vi "PointsToROI.vi"(11 "Points":dbl[][](array[numeric])) -> (3 "ROIs":T1(array[cluster]))   [LabVIEW 2012]
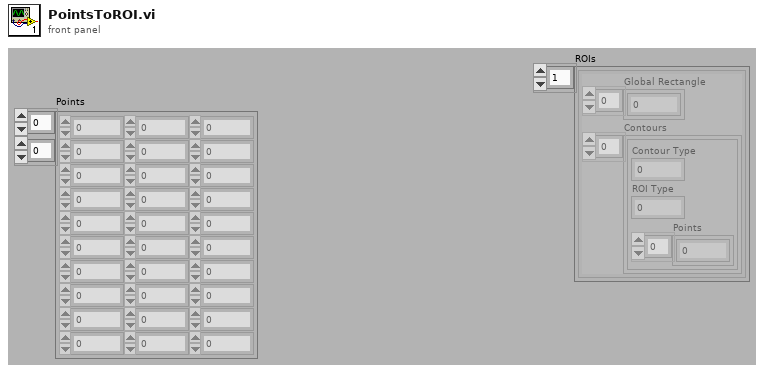
[diagram p1: front panel]
types:
  T1 = cluster{"Global Rectangle":i32[], "Contours":cluster{"Contour Type":u32, "ROI Type":u32, "Points":i32[]}[]}[]
  T2 = cluster{"Global Rectangle":i32[], "Contours":cluster{"Contour Type":u32, "ROI Type":u32, "Points":i32[]}[]}
  T3 = cluster{"Contour Type":u32, "ROI Type":i32, "Points":i32[]}
  T4 = cluster{"Contour Type":u32, "ROI Type":u32, "Points":i32[]}[]
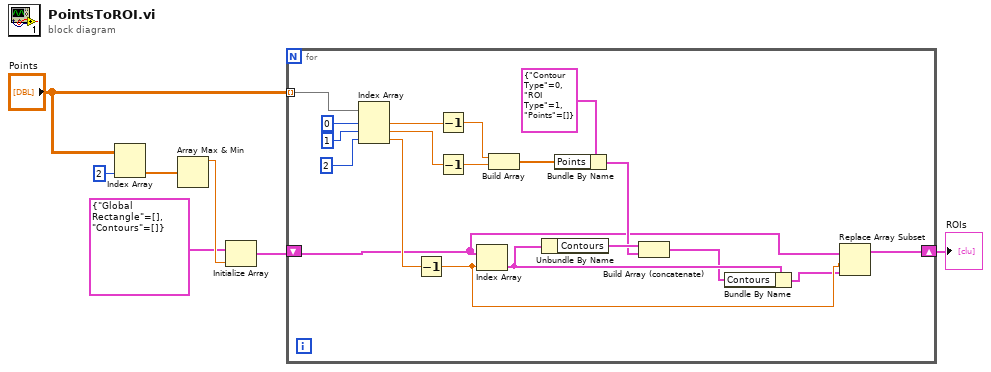
[diagram p0: block diagram]
diagram:
  n1 = Index Array(array="Points", index (col)=2 ("disabled index (col)")) -> (element=w6:dbl[])  [unwired: 1 in]
  n2 = Array Max & Min(array=w6) -> (max value=w5:dbl)  [unwired: 3 out]
  n3 = Initialize Array(T2 {"Global Rectangle"=[], "Contours"=[]} ("ROI"), w5) -> (w2:T1)
  n4 = for {
    tunnel: "Points" -> [w26] mode=indexing
    shift-right: [w14] -> w1
    shift-left: w2 -> [w18]
    n5 = Index Array(array=w26, index #1=0 ("index"), index #2=1 ("index"), index #3=2 ("index")) -> (element #1=w9:dbl, element #2=w11:dbl, element #3=w24:dbl)
    n6 = Decrement(x=w24) -> (x-1=w17:dbl)
    n7 = Decrement(x=w9) -> (x-1=w8:dbl)
    n8 = Decrement(x=w11) -> (x-1=w10:dbl)
    n9 = Index Array(array=w18, index=w17) -> (element=w22:T2)
    n10 = Build Array(w8, w10) -> (w15:dbl[])
    n11 = Unbundle By Name(w22) -> ("Contours"=w23:T4)
    n12 = Bundle By Name(cluster=T3 {"Contour Type"=0, "ROI Type"=1, "Points"=[]}, "Points"=w15) -> (w19:T3)
    n13 = Build Array (concatenate)(w23, w19) -> (w21:T4)
    n14 = Bundle By Name(cluster=w22, "Contours"=w21) -> (w16:T2)
    n15 = Replace Array Subset(array=w18, new element=w16, index=w17) -> (w14:T1)
  }
  "ROIs" <- w1
